vi "Calibrate.vi"(11 "Calculated Vertical Angle":dbl) -> (3 "Vertical Angle Error":dbl)   [LabVIEW 2011]
panel:
  in  "Dist in Ft":dbl=21.1666
  in  "Diff in Height":dbl=52.5
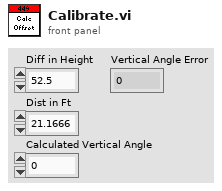
[diagram p1: front panel]
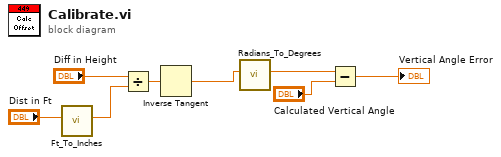
[diagram p0: block diagram]
diagram:
  n1 = call "Ft_To_Inches.vi"("Ft"="Dist in Ft") -> ("In"=w5:dbl)  [unwired: 10 in]
  n2 = Divide(x="Diff in Height", y=w5) -> (x/y=w6:dbl)
  n3 = Inverse Tangent(1:w6) -> (0:w4:dbl)
  n4 = call "Radians_To_Degrees.vi"("Radians"=w4) -> ("Degrees"=w3:dbl)  [unwired: 10 in]
  n5 = Subtract(x=w3, y="Calculated Vertical Angle") -> (x-y=→"Vertical Angle Error":dbl)
